vi "Logging.vi"(8 "error in (no error)":errorcluster caption="错误输入（无错误）", 10 "Log":string, 11 "Log 输入":refnum<class "Log.lvclass">) -> (0 "error out":errorcluster caption="错误输出", 3 "Log 输出":refnum<class "Log.lvclass">)   [LabVIEW 2019, in "Log.lvlib" / "Log.lvclass"]
uses:
  Log.lvclass
  Log.lvclass/Log.ctl
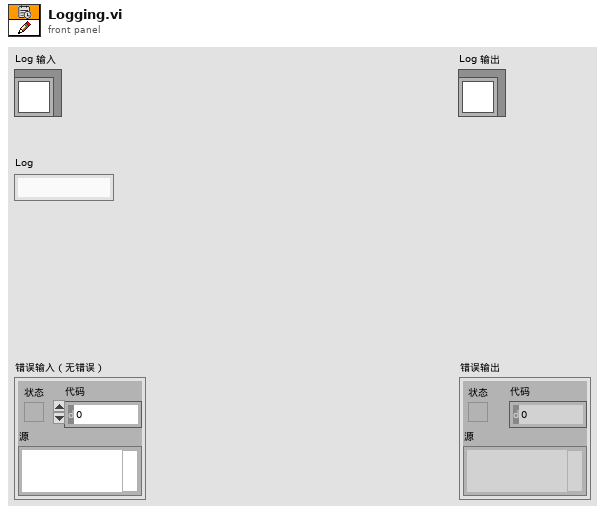
[diagram p1: front panel]
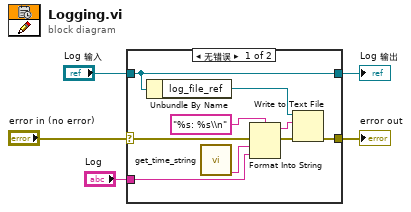
[diagram p0: block diagram]
diagram:
  n1 = case shown="无错误" "error in (no error)" {
    selector: "error in (no error)" -> [w9 w16]
    tunnel: [w7 w16] -> w4
    tunnel: [w11 w15] -> w2
    tunnel: "Log 输入" -> [w11 w15]
    tunnel: "Log" -> [w12 _]
    frame No Error {
      n2 = Unbundle By Name(w11) -> ("log_file_ref"=w8:refnum<file>)
      n3 = call "get_time_string.vi"() -> ("date/time string"=w13:string)  [unwired: 11 in]
      n4 = Format Into String(format string="%s: %s\\n" ("格式字符串"), error in=w9, w13, w12) -> (resulting string=w6:string, error out=w10:errorcluster)  [unwired: 1 in]
      n5 = Write to Text File(file (use dialog)=w8, text=w6, error in=w10) -> (error out=w7:errorcluster)  [unwired: 1 in, 2 out]
    }
    frame Error {
    }
  }
  "error out" <- w4
  "Log 输出" <- w2
